vi "Event Handler.vi"(8 "error in (no error)":errorcluster, 10 "Stop Event Handler":refnum<user-event>, 11 "SingleStepTestV3 in":refnum<class "SingleStepTestV2.lvclass">) -> (0 "error out":errorcluster)   [LabVIEW 2016, in "SingleStepTestV2.lvlib" / "SingleStepTestV2.lvclass"]
doc: "The <b>Event Handler VI</b> is a dynamic dispatch VI that should be overwritten if events are needed to create the enhanced QControl. \n\nBy inheriting from the main Control.lvclass the overwritten <b>Event Handler VI</b> will be launched asynchronously in the initialization of the QControl.\n<b> </b> <b> </b>\n©2016 Q Software Innovations, LLC (QSI)\nwritten by Quentin Alldredge\nproduced in LabVIEW 2015\n\nsupport@qsoftwareinnovations.com\nwww.qsoftwareinnovations.com\n\nAll rights reserved.\n\nRedistribution and use in source and binary forms, with or without modification, are permitted provided that the following conditions are met:\n\n * Redistributions of source code must retain the above copyright notice, this list of conditions and the following disclaimer.\n * Redistributions in binary form must reproduce the above copyright notice, this list of conditions and the following disclaimer in the documentation and/or other materials provided with the distribution.\n * Neither the name of Q Software Innovations, LLC. nor the names of its contributors may be used to endorse or promote products derived from this software without specific prior written permission.\n\nTHIS SOFTWARE IS PROVIDED BY THE COPYRIGHT HOLDERS AND CONTRIBUTORS \"AS IS\" AND ANY EXPRESS OR IMPLIED WARRANTIES, INCLUDING, BUT NOT LIMITED TO, THE IMPLIED WARRANTIES OF MERCHANTABILITY AND FITNESS FOR A PARTICULAR PURPOSE ARE DISCLAIMED. IN NO EVENT SHALL THE COPYRIGHT OWNER OR CONTRIBUTORS BE LIABLE FOR ANY DIRECT, INDIRECT, INCIDENTAL, SPECIAL, EXEMPLARY, OR CONSEQUENTIAL DAMAGES (INCLUDING, BUT NOT LIMITED TO, PROCUREMENT OF SUBSTITUTE GOODS OR SERVICES; LOSS OF USE, DATA, OR PROFITS; OR BUSINESS INTERRUPTION) HOWEVER CAUSED AND ON ANY THEORY OF LIABILITY, WHETHER IN CONTRACT, STRICT LIABILITY, OR TORT (INCLUDING NEGLIGENCE OR OTHERWISE) ARISING IN ANY WAY OUT OF THE USE OF THIS SOFTWARE, EVEN IF ADVISED OF THE POSSIBILITY OF SUCH DAMAGE."
uses:
  SingleStepTestV2.lvclass
  SingleStepTestV2.lvclass/SingleStepTestV2.ctl
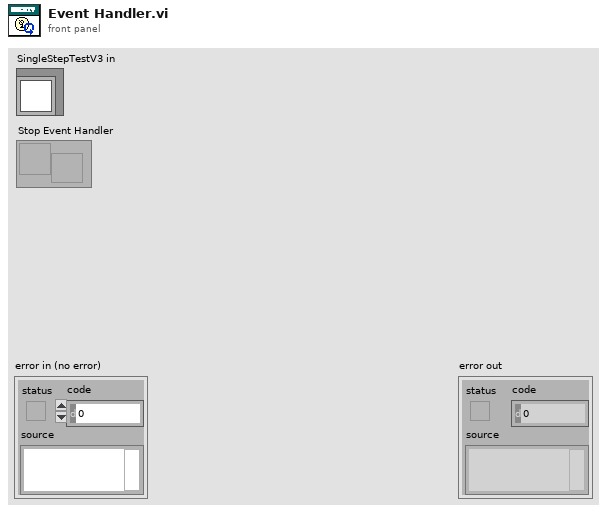
[diagram p1: front panel]
types:
  T1 = typedef "SingleStepTestV2.lvclass/注射泵操作.ctl" = enum32{"复位", "注入", "注出", "等待"}
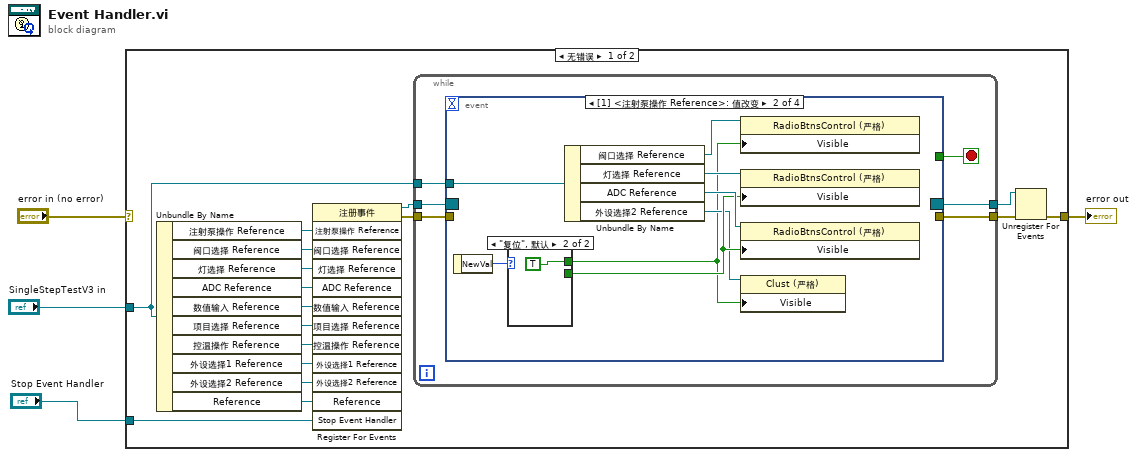
[diagram p0: block diagram]
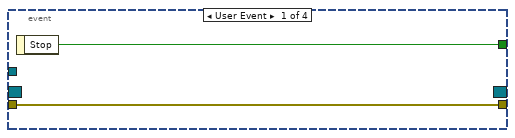
[diagram p2: hidden frame]
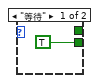
[diagram p3: hidden frame]
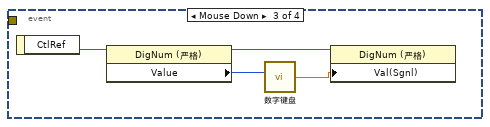
[diagram p4: hidden frame]
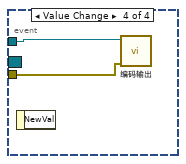
[diagram p5: hidden frame]
diagram:
  n1 = case shown="无错误" "error in (no error)" {
    selector: "error in (no error)" -> [_ w46]
    tunnel: [w18 w46] -> w3
    tunnel: "SingleStepTestV3 in" -> [w16 _]
    tunnel: "Stop Event Handler" -> [w15 _]
    frame No Error {
      n2 = Unbundle By Name(w16) -> ("注射泵操作 Reference"=w14:refnum<vi>, "阀口选择 Reference"=w13:refnum<vi>, "灯选择 Reference"=w12:refnum<vi>, "ADC Reference"=w11:refnum<vi>, "数值输入 Reference"=w10:refnum<vi>, "项目选择 Reference"=w9:refnum<vi>, "控温操作 Reference"=w8:refnum<vi>, "外设选择1 Reference"=w7:refnum<vi>, "外设选择2 Reference"=w6:refnum<vi>, "Reference"=w5:refnum<vi>)
      n3 = register-events(w14, w13, w12, w11, w10, w9, w8, w7, w6, w5, w15) -> (reference out=w21:refnum<event-registration>, error out=w20:errorcluster)  [unwired: 2 in]
      n4 = while {
        tunnel: w21 -> [w27]
        tunnel: w20 -> [w25]
        tunnel: [w24] -> w19
        tunnel: [w22] -> w17
        tunnel: w16 -> [w26]
        stop <- w23 stop-if-true
        n5 = event shown="[1] <注射泵操作 Reference>: 值改变" {
          selector: w27 -> [_ _ _ _]
          dyn-events: [_ _ _ _] -> w22
          timeout: _ -> [_ _ _ _]
          tunnel: w26 -> [_ w37 _ w45]
          tunnel: w25 -> [w29 _ _ w44]
          tunnel: [w29 _ _ _] -> w24
          tunnel: [w28 _ _ _] -> w23
          event User Event {
            n6 = event-data() -> ("Stop"=w28:bool)  [unwired: 1 in]
          }
          event Value Change {
            n7 = event-data() -> ("NewVal"=w36:T1)  [unwired: 1 in]
            n8 = case shown="\"复位\", 默认" w36 {
              tunnel: [TRUE _] -> w32
              tunnel: [_ TRUE] -> w30
              frame "等待" {
              }
              frame "复位", Default {
              }
            }
            n9 = Unbundle By Name(w37) -> ("阀口选择 Reference"=w35:refnum<vi>, "灯选择 Reference"=w34:refnum<vi>, "ADC Reference"=w33:refnum<vi>, "外设选择2 Reference"=w31:refnum<vi>)
            n10 = property class="RadioBtnsControl (严格)"(reference=w35, "Visible"=w30) -> ()  [unwired: 1 in, 2 out]
            n11 = property class="RadioBtnsControl (严格)"(reference=w34, "Visible"=w32) -> ()  [unwired: 1 in, 2 out]
            n12 = property class="RadioBtnsControl (严格)"(reference=w33, "Visible"=w32) -> ()  [unwired: 1 in, 2 out]
            n13 = property class="Clust (严格)"(reference=w31, "Visible"=w30) -> ()  [unwired: 1 in, 2 out]
          }
          event Mouse Down {
            n14 = event-data() -> ("CtlRef"=w43:refnum<vi>)  [unwired: 1 in]
            n15 = property class="DigNum (严格)"(reference=w43) -> (reference out=w41:refnum<vi>, "Value"=w42:i16)  [unwired: 1 in, 1 out]
            n16 = call "数字键盘.vi"("OldNumber"=w42) -> ("NewNumber"=w40:sgl)
            n17 = property class="DigNum (严格)"(reference=w41, "Val(Sgnl)"=w40) -> ()  [unwired: 1 in, 2 out]
          }
          event Value Change {
            n18 = event-data() -> ()  [unwired: 1 in, 1 out]
            n19 = call "编码输出.vi"("error in (no error)"=w44, "SingleStepTestV3输入"=w45) -> ()  [unwired: 9 in, 1 out]
          }
        }
      }
      n20 = Unregister For Events(event registration refnum=w17, error in=w19) -> (error out=w18:errorcluster)
    }
    frame Error {
    }
  }
  "error out" <- w3
